vi "Cathode_controller_tb.vi"() -> ()   [LabVIEW 2018]
uses:
  Global Stop.vi
panel:
  out "Waveform Chart":dbl(graph)
  out "PS 1 Output Voltage":dbl
  in  "stop":bool
  in  "Relay 3":dbl
  in  "Relay 2":dbl
  in  "Relay 1":dbl
  in  "Thermocouple":dbl(slide) scale=0.0..2000.0
  out "Temperture display":dbl(slide) scale=0.0..2000.0
  in  "Voltage set":dbl
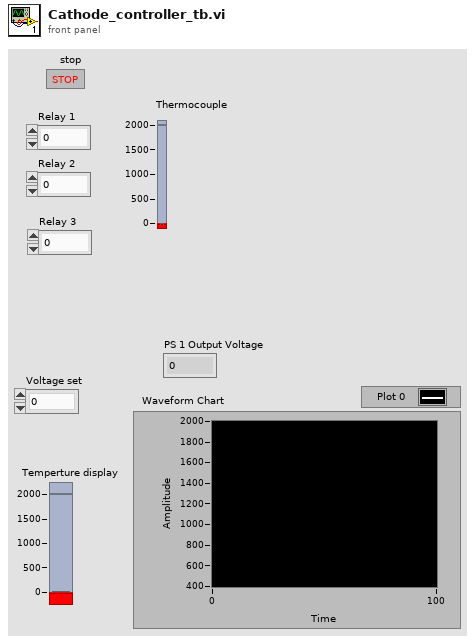
[diagram p1: front panel]
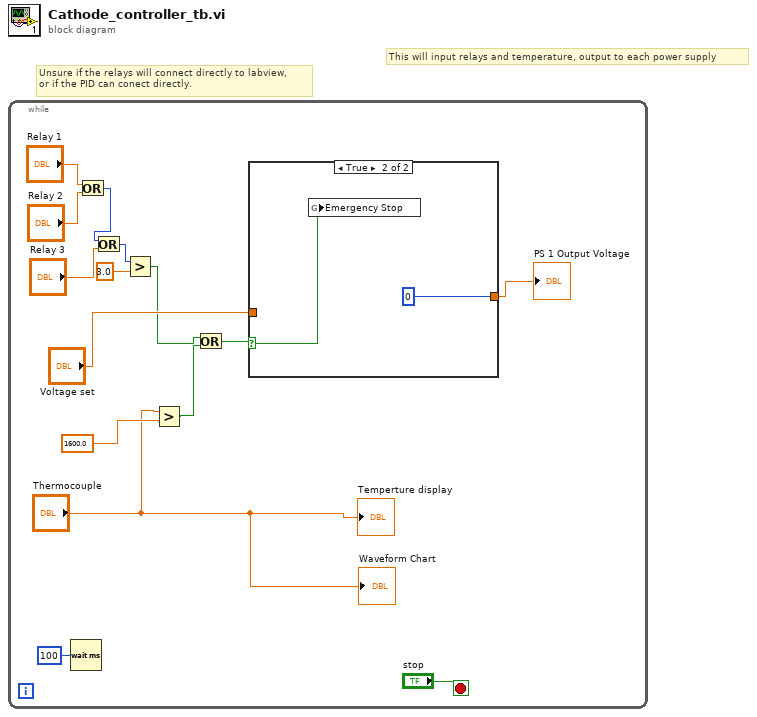
[diagram p0: block diagram]
diagram:
  # "Unsure if the relays will connect directly to labview, \nor if the PID can conect directly."
  # "This will input relays and temperature, output to each power supply"
  n1 = while {
    stop <- "stop" stop-if-true
    n2 = Wait (ms)(milliseconds to wait=u32 100) -> ()  [unwired: 1 out]
    n3 = Or(x="Relay 1", y="Relay 2") -> (x .or. y?=w11:i32)
    n4 = Or(x=w11, y="Relay 3") -> (x .or. y?=w8:i32)
    n5 = Greater?(x=w8, y=3.0) -> (0:w5:bool)
    n6 = Greater?(x="Thermocouple", y=1600.0) -> (0:w3:bool)
    n7 = Or(x=w5, y=w3) -> (x .or. y?=w4:bool)
    n8 = case shown="True" w4 {
      selector: w4 -> [_ w18]
      tunnel: [w16 0] -> w6
      tunnel: "Voltage set" -> [w16 _]
      frame False {
      }
      frame True {
        n9 = global write "Global Stop.vi" "Emergency Stop"(w18) -> ()
      }
    }
    "PS 1 Output Voltage" <- w6
    "Temperture display" <- "Thermocouple"
    "Waveform Chart" <- "Thermocouple"
  }
